vi "Configure Trigger (SPI).vi"(0 "VISA resource name":refnum<visa-resource-name>, 5 "Trigger Source (9: Bus 1)":u16(ring)=9 items=["Bus 1"=9, "Bus 2"=10, "Bus 3"=11, "Bus 4"=12], 7 "Trigger Condition (0: SS)":u16(ring) items=["SS", "Start of Frame", "MISO", "MOSI", "MISO & MOSI"], 9 "MISO & MOSI":T1={"Data Size (1)"=1, "MISO Value"="XXXXXXXX", "MOSI Value"="XXXXXXXX"}, 11 "error in (no error)":errorcluster) -> (4 "VISA resource name out":refnum<visa-resource-name>, 15 "error out":errorcluster)   [LabVIEW 2009, in "Tektronix DPO MSO 2000 4000 Series.lvlib"]
doc: "Configures SPI trigger settings for an oscilloscope."
uses:
  <instrlib>/Tektronix DPO MSO 2000 4000 Series/Tektronix DPO MSO 2000 4000 Series.lvlib
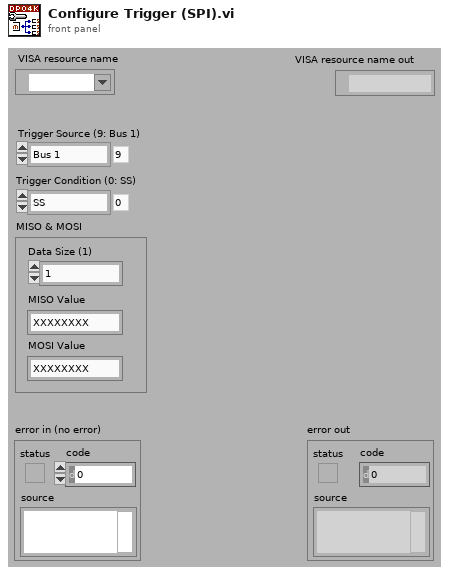
[diagram p1: front panel]
types:
  T1 = cluster{"Data Size (1)":i32, "MISO Value":string, "MOSI Value":string}
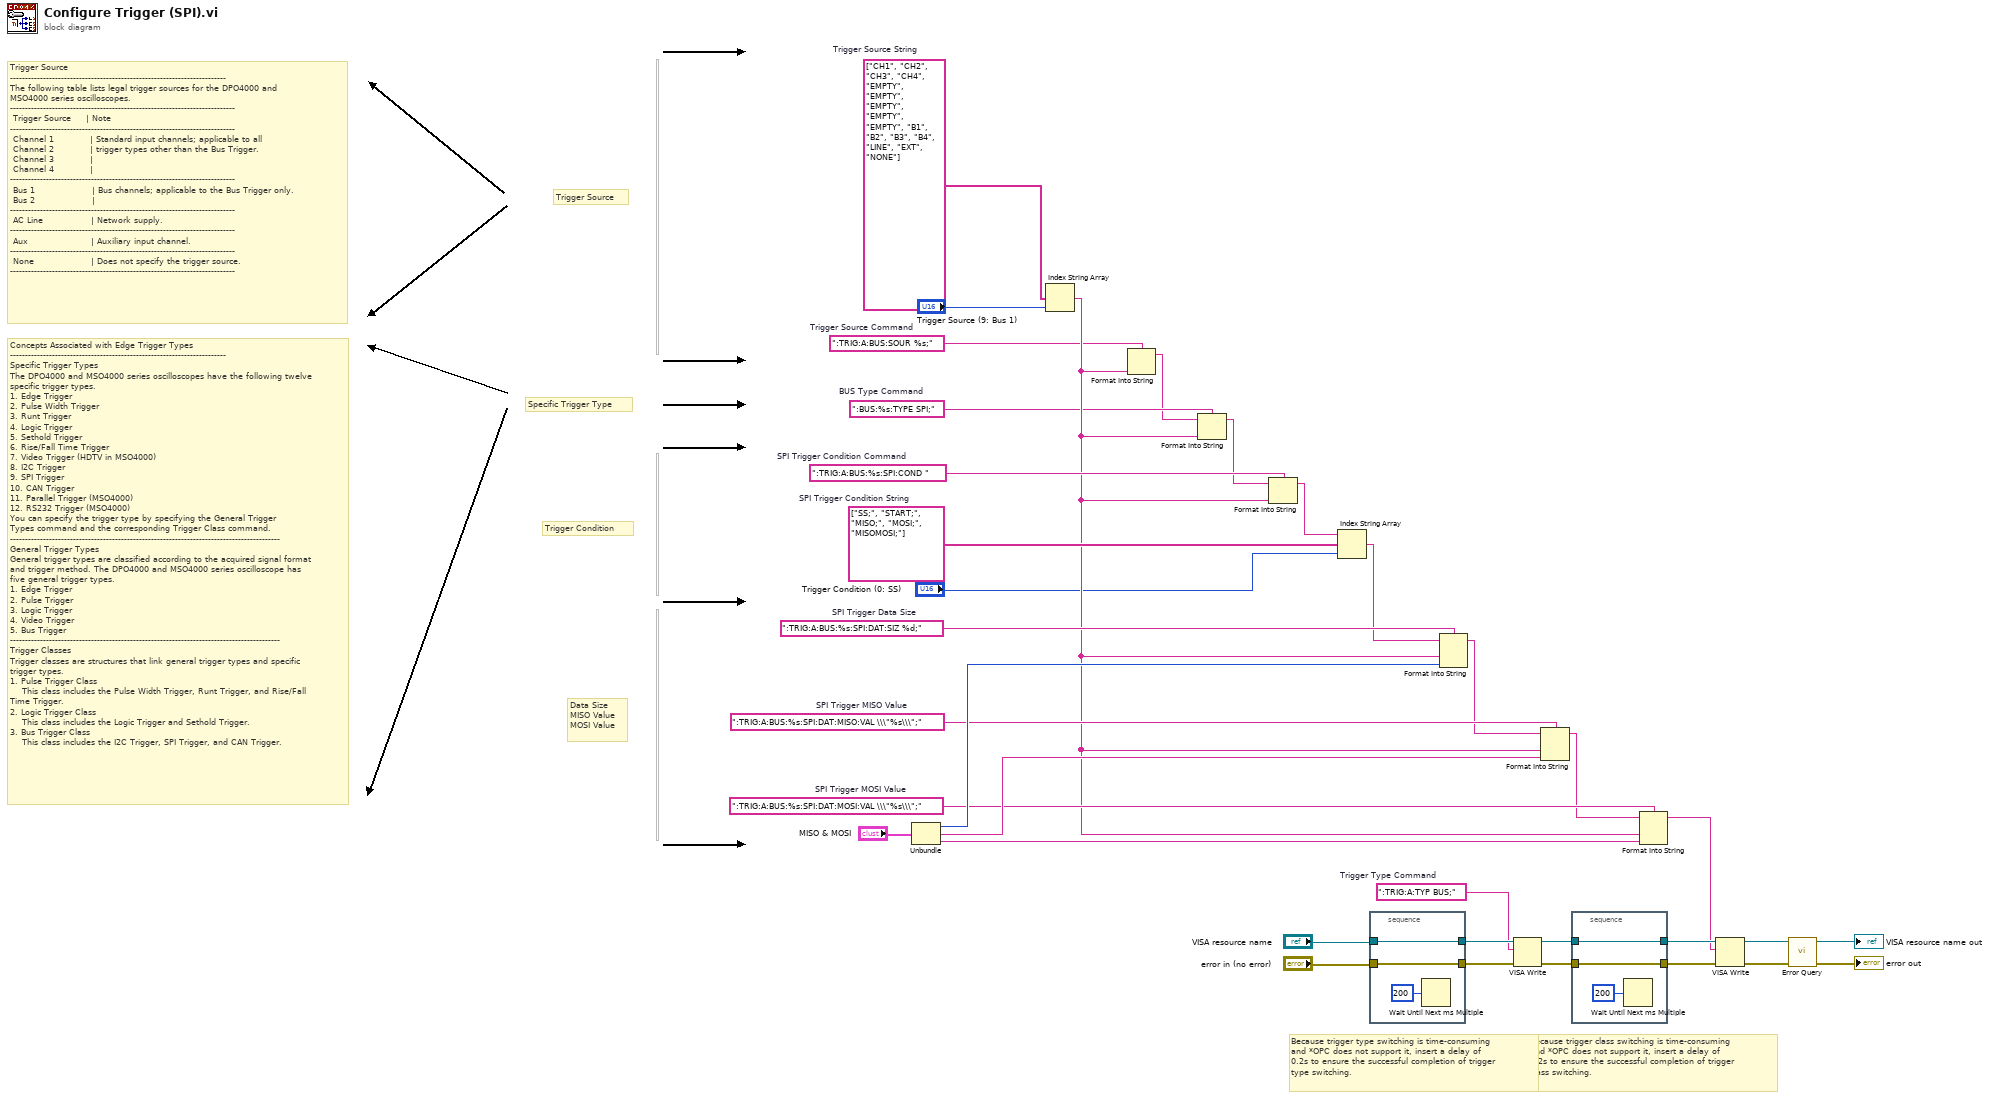
[diagram p0: block diagram]
diagram:
  w19 = string[] ["CH1", "CH2", "CH3", "CH4", "EMPTY", "EMPTY", "EMPTY", "EMPTY", "EMPTY", "B1", "B2", "B3", "B4", "LINE", "EXT", "NONE"]  # Trigger Source String
  w13 = ":TRIG:A:BUS:SOUR %s;"  # Trigger Source Command
  w24 = ":TRIG:A:TYP BUS;"  # Trigger Type Command
  w27 = ":TRIG:A:BUS:%s:SPI:DAT:MOSI:VAL \\\"%s\\\";"  # SPI Trigger MOSI Value
  w28 = ":TRIG:A:BUS:%s:SPI:DAT:MISO:VAL \\\"%s\\\";"  # SPI Trigger MISO Value
  w32 = ":TRIG:A:BUS:%s:SPI:DAT:SIZ %d;"  # SPI Trigger Data Size
  w34 = string[] ["SS;", "START;", "MISO;", "MOSI;", "MISOMOSI;"]  # SPI Trigger Condition String
  w35 = ":TRIG:A:BUS:%s:SPI:COND "  # SPI Trigger Condition Command
  w14 = ":BUS:%s:TYPE SPI;"  # BUS Type Command
  # "Concepts Associated with Edge Trigger Types\n------------------------------------------------------------------------\nSpecific Trigger Types\nThe DPO4000 and MSO4000 series oscilloscopes have the following twelve specific trigger types.\n1. Edge Trigger\n2. Pulse Width Trigger\n3. Runt Trigger\n4. Logic Trigger\n5. Sethold Trigger\n6. Rise/Fall Time Trigger\n7. Video Trigger (HDTV in MSO4000)\n8. I2C Trigger\n9. SPI Trigger\n10. CAN Trigger\n11. Parallel Trigger (MSO4000)\n12. RS232 Trigger (MSO4000)\nYou can specify the trigger type by specifying the General Trigger \nTypes command and the corresponding Trigger Class command.\n------------------------------------------------------------------------------------------\nGeneral Trigger Types \nGeneral trigger types are classified according to the acquired signal format and trigger method. The DPO4000 and MSO4000 series oscilloscope has five general trigger types.\n1. Edge Trigger\n2. Pulse Trigger\n3. Logic Trigger\n4. Video Trigger\n5. Bus Trigger\n------------------------------------------------------------------------------------------\nTrigger Classes\nTrigger classes are structures that link general trigger types and specific trigger types.\n1. Pulse Trigger Class\n    This class includes the Pulse Width Trigger, Runt Trigger, and Rise/Fall Time Trigger.\n2. Logic Trigger Class\n    This class includes the Logic Trigger and Sethold Trigger.\n3. Bus Trigger Class\n    This class includes the I2C Trigger, SPI Trigger, and CAN Trigger."
  # "Trigger Source\n------------------------------------------------------------------------\nThe following table lists legal trigger sources for the DPO4000 and MSO4000 series oscilloscopes.\n---------------------------------------------------------------------------\n Trigger Source     | Note                                                           \n---------------------------------------------------------------------------\n Channel 1            | Standard input channels; applicable to all      \n Channel 2            | trigger types other than the Bus Trigger.         \n Channel 3            |     \n Channel 4            |\n---------------------------------------------------------------------------\n Bus 1                   | Bus channels; applicable to the Bus Trigger only.\n Bus 2                   | \n---------------------------------------------------------------------------\n AC Line                | Network supply.\n---------------------------------------------------------------------------\n Aux                     | Auxiliary input channel.\n---------------------------------------------------------------------------\n None                   | Does not specify the trigger source.\n---------------------------------------------------------------------------"
  # "Because trigger class switching is time-consuming\nand *OPC does not support it, insert a delay of\n0.2s to ensure the successful completion of trigger\nclass switching."
  # "Because trigger type switching is time-consuming\nand *OPC does not support it, insert a delay of\n0.2s to ensure the successful completion of trigger\ntype switching."
  # "Data Size\nMISO Value\nMOSI Value"
  # "Trigger Condition"
  # "Specific Trigger Type"
  # "Trigger Source"
  n1 = Unbundle("MISO & MOSI") -> ("Data Size (1)"=w29:i32, "MISO Value"=w31:string, "MOSI Value"=w30:string)
  n2 = Index String Array(1:"Trigger Source (9: Bus 1)", 2:w19) -> (0:w18:string)  [unwired: 1 in]
  n3 = Format Into String(format string=w13, w18) -> (resulting string=w9:string)  [unwired: 2 in, 1 out]
  n4 = Format Into String(format string=w14, initial string=w9, w18) -> (resulting string=w12:string)  [unwired: 1 in, 1 out]
  n5 = Format Into String(format string=w35, initial string=w12, w18) -> (resulting string=w33:string)  [unwired: 1 in, 1 out]
  n6 = Index String Array(1:"Trigger Condition (0: SS)", 2:w34, 3:w33) -> (0:w11:string)
  n7 = stacked-sequence {
    tunnel: "VISA resource name" -> [w37]
    tunnel: [w37] -> w26
    tunnel: "error in (no error)" -> [w36]
    tunnel: [w36] -> w25
    frame #0 {
      n8 = Wait Until Next ms Multiple(millisecond multiple=u32 200) -> ()  [unwired: 1 out]
    }
  }
  n9 = Format Into String(format string=w32, initial string=w11, w18, w29) -> (resulting string=w8:string)  [unwired: 1 in, 1 out]
  n10 = VISA Write(VISA resource name=w26, write buffer=w24, error in (no error)=w25) -> (VISA resource name out=w23:refnum<visa-resource-name>, error out=w22:errorcluster)  [unwired: 1 out]
  n11 = Format Into String(format string=w28, initial string=w8, w18, w31) -> (resulting string=w10:string)  [unwired: 1 in, 1 out]
  n12 = stacked-sequence {
    tunnel: w23 -> [w40]
    tunnel: [w40] -> w21
    tunnel: w22 -> [w39]
    tunnel: [w39] -> w20
    frame #0 {
      n13 = Wait Until Next ms Multiple(millisecond multiple=u32 200) -> ()  [unwired: 1 out]
    }
  }
  n14 = Format Into String(format string=w27, initial string=w10, w18, w30) -> (resulting string=w7:string)  [unwired: 1 in, 1 out]
  n15 = VISA Write(VISA resource name=w21, write buffer=w7, error in (no error)=w20) -> (VISA resource name out=w6:refnum<visa-resource-name>, error out=w5:errorcluster)  [unwired: 1 out]
  n16 = call <instrlib>:"Error Query.vi"("error in (no error)"=w5, "VISA resource name"=w6) -> ("error out"=→"error out":errorcluster, "VISA resource name out"=→"VISA resource name out":refnum<visa-resource-name>)  [unwired: 6 in, 2 out]
